vi "Exit recursion.vi"(0 "combo index in":i32, 1 "Iterations array in":i32[](array[numeric]), 2 "Quantities":i32[](array[numeric]), 5 "Combos in":i32[][](array[numeric]), 7 "Values":i32[](array[numeric]), 9 "Goal amount":i32, 11 "Depth":i32, 12 "Result index in":i32, 13 "Results in":i32[][](array[numeric])) -> (4 "Progress - current iteration values":i32[](array[numeric]), 6 "Combo index out":i32, 8 "Combos out":i32[][](array[numeric]), 10 "Result index out":i32, 14 "Results out":i32[][](array[numeric]))   [LabVIEW 2018]
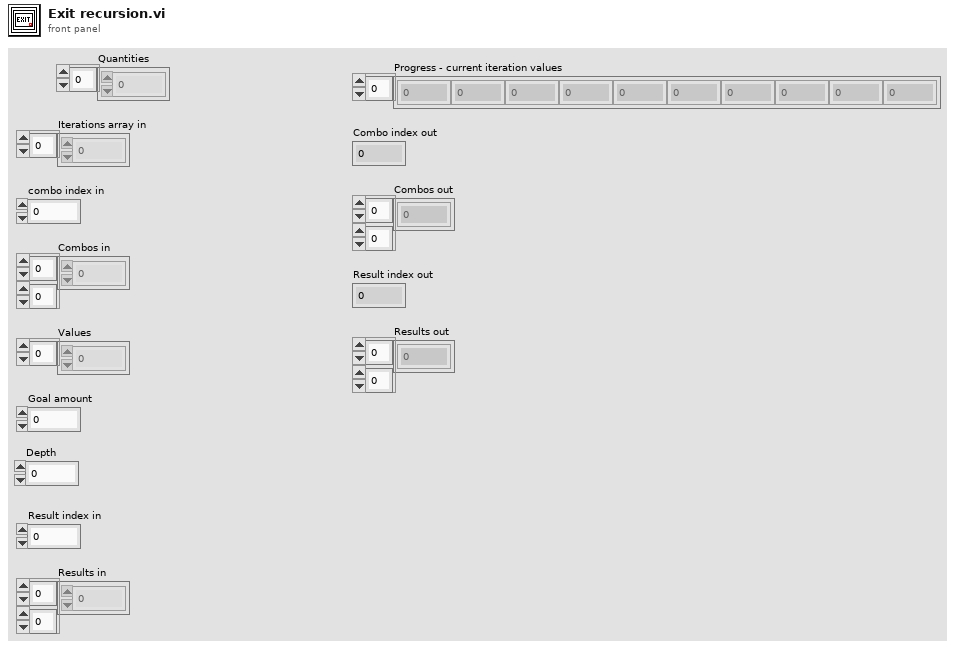
[diagram p1: front panel]
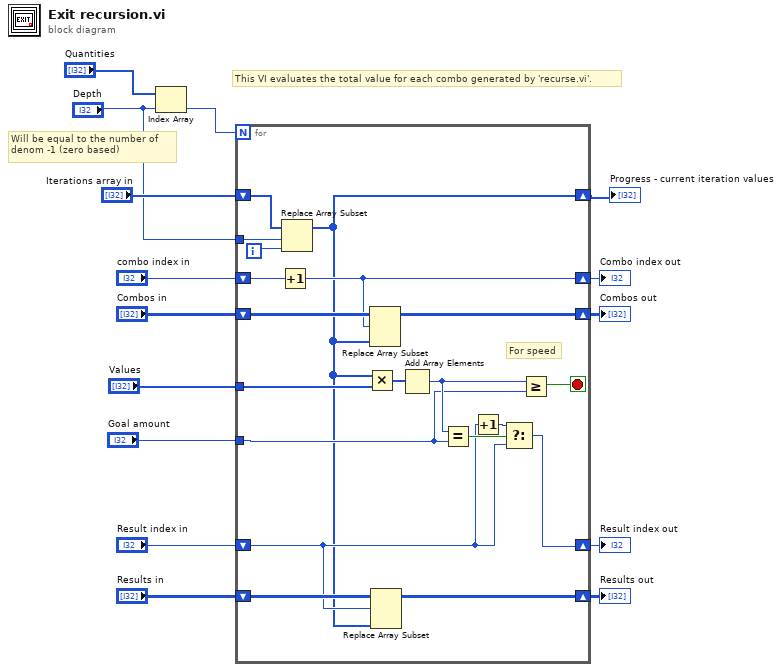
[diagram p0: block diagram]
diagram:
  # "Will be equal to the number of \ndenom -1 (zero based)"
  # "This VI evaluates the total value for each combo generated by 'recurse.vi'."
  n1 = Index Array(array="Quantities", index="Depth") -> (element=w3:i32)
  n2 = for {
    N: w3 -> [_]
    shift-right: [w33] -> w5
    shift-left: "Combos in" -> [w34]
    shift-right: [w31] -> w8
    shift-left: "combo index in" -> [w32]
    tunnel: "Values" -> [w29]
    shift-right: [w26] -> w13
    shift-left: "Result index in" -> [w23]
    shift-right: [w25] -> w12
    shift-left: "Results in" -> [w24]
    shift-right: [w16] -> w2
    shift-left: "Iterations array in" -> [w17]
    tunnel: "Goal amount" -> [w20]
    tunnel: "Depth" -> [w18]
    i -> [w19]
    stop <- w21 stop-if-true
    # "For speed"
    n3 = Increment(x=w32) -> (x+1=w31:i32)
    n4 = Replace Array Subset(array=w17, new element=w19, index=w18) -> (w16:i32[])
    n5 = Multiply(x=w16, y=w29) -> (x*y=w30:i32[])
    n6 = Replace Array Subset(array=w34, new element=w16, index (row)=w31) -> (w33:i32[][])  [unwired: 1 in]
    n7 = Replace Array Subset(array=w24, new element=w16, index (row)=w23) -> (w25:i32[][])  [unwired: 1 in]
    n8 = Add Array Elements(numeric array=w30) -> (sum=w22:i32)
    n9 = Equal?(x=w22, y=w20) -> (x = y?=w28:bool)
    n10 = Increment(x=w23) -> (x+1=w27:i32)
    n11 = Select(t=w27, s=w28, f=w23) -> (s? t:f=w26:i32)
    n12 = Greater Or Equal?(x=w22, y=w20) -> (x >= y?=w21:bool)
  }
  "Result index out" <- w13
  "Results out" <- w12
  "Combo index out" <- w8
  "Combos out" <- w5
  "Progress - current iteration values" <- w2
